vi "1553B_帧解析_v4_27.vi"(8 "ZhuBeiFen?":string="Zhufen_period", 9 "Counter":u64, 11 "数组":u8[](array[numeric])) -> (1 "连接的字符串":string, 3 "输出簇":T1)   [LabVIEW 2012]
uses:
  <vilib>/GPower/VIRegister/Library/Convert/ToU16.vi
  <vilib>/GPower/VIRegister/Library/SubVIs/FindRegisterData.vi
  <vilib>/GPower/VIRegister/Library/SubVIs/ReadSub.vi
  <vilib>/GPower/VIRegister/Library/QManager/GetRegisterData.vi
  <vilib>/GPower/Error/Library/SetError.vi
  <vilib>/GPower/Error/Library/FilterCodes.vi
  <vilib>/GPower/Error/Library/Filter/FilterMulti.vi
  <vilib>/GPower/VIRegister/Library/QManager/QManagerAction.vi
  <vilib>/GPower/Error/Library/ErrorType.vi
  <vilib>/GPower/Error/Library/SplitAppended.vi
  <vilib>/GPower/Error/Library/SubVIs/ExplanationToError.vi
  <vilib>/GPower/VIRegister/Library/QManager/GetQName.vi
  <vilib>/GPower/VIRegister/Library/QManager/StartQManager.vi
  <vilib>/Utility/error.llb/Trim Whitespace.vi
  <vilib>/dlg_ctls.llb/Space Constant.vi
  <vilib>/Utility/error.llb/Error Code Database.vi
  <vilib>/GPower/Error/Library/SubVIs/SetStatus.vi
  <vilib>/GPower/Error/Library/AppendErrors.vi
  <vilib>/GPower/Error/Library/Append/AppendSingle.vi
  <vilib>/GPower/VIRegister/VIRegister.lvlib
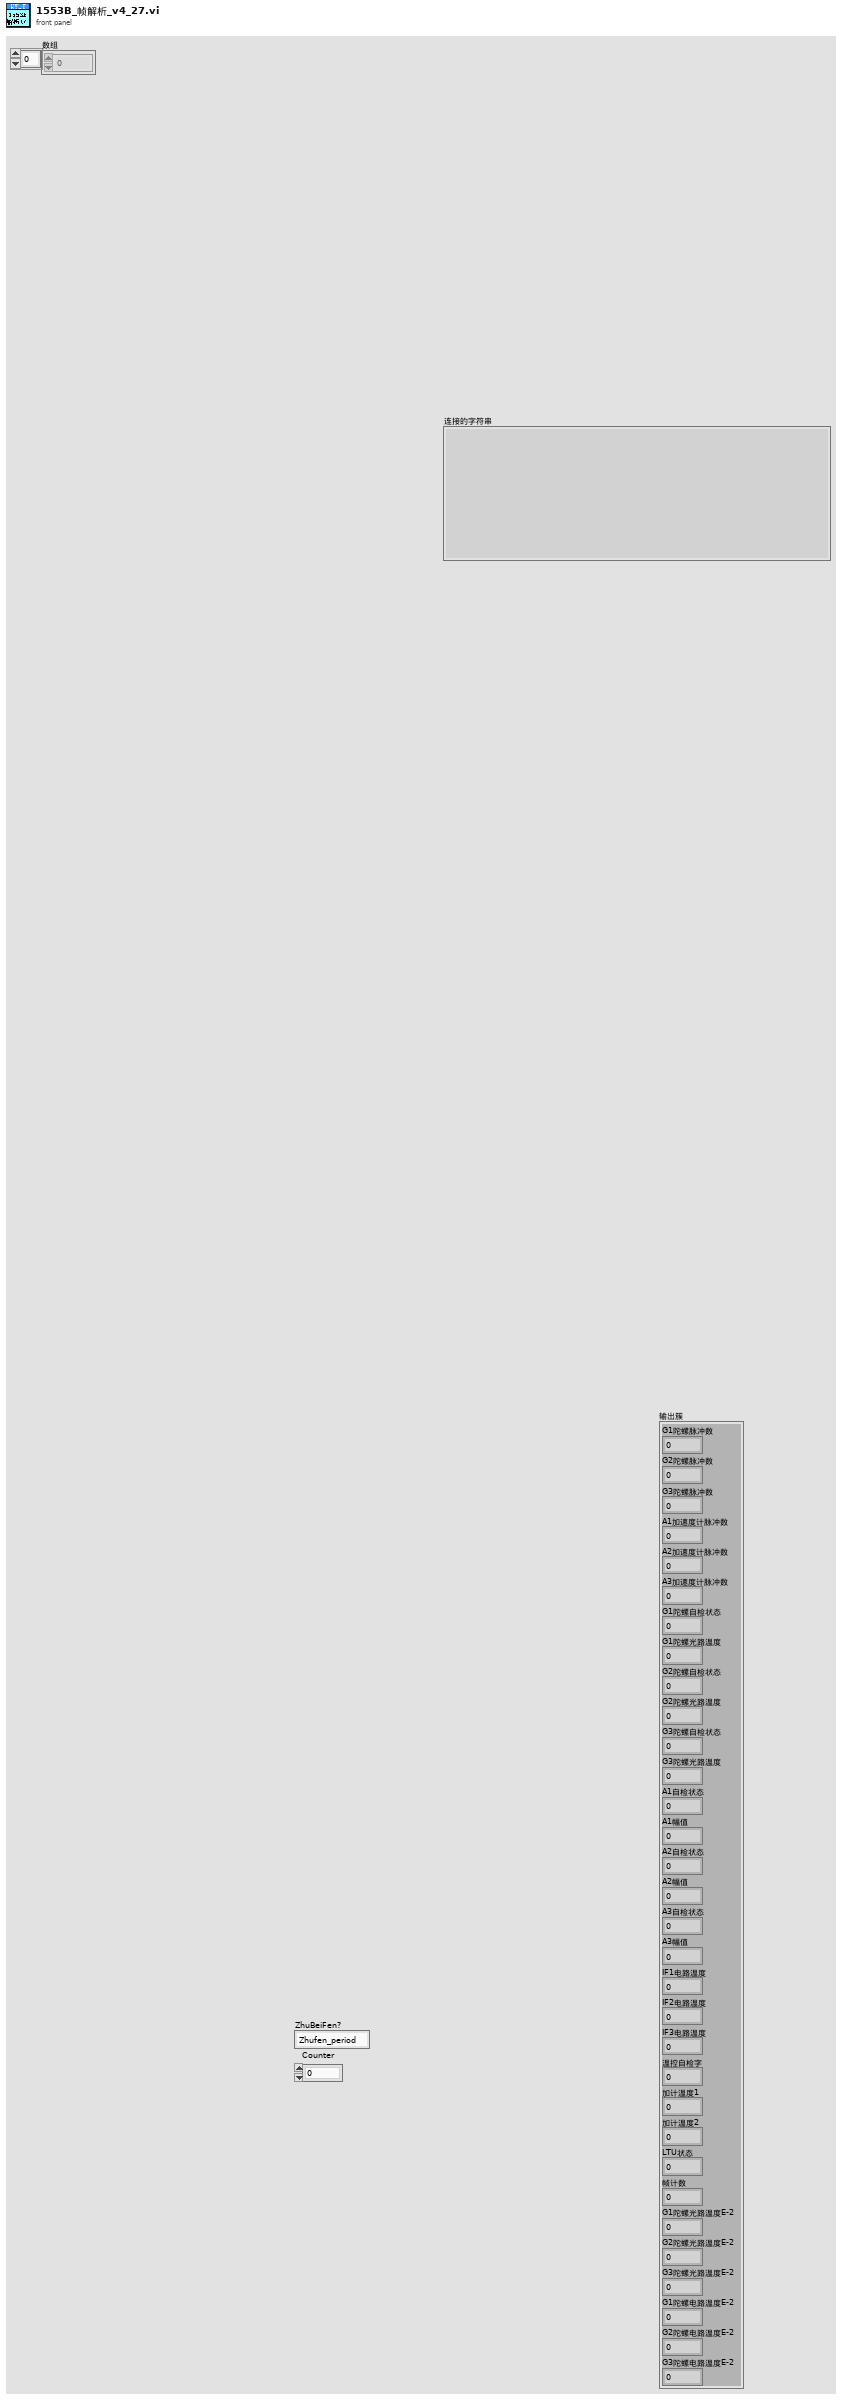
[diagram p1: front panel]
types:
  T1 = cluster{"G1陀螺脉冲数":i32, "G2陀螺脉冲数":i32, "G3陀螺脉冲数":i32, "A1加速度计脉冲数":i16, "A2加速度计脉冲数":i16, "A3加速度计脉冲数":i16, "G1陀螺自检状态":u8, "G1陀螺光路温度":i8, "G2陀螺自检状态":u8, "G2陀螺光路温度":i8, "G3陀螺自检状态":u8, "G3陀螺光路温度":i8, "A1自检状态":u8, "A1幅值":u8, "A2自检状态":u8, "A2幅值":u8, "A3自检状态":u8, "A3幅值":u8, "IF1电路温度":i8, "IF2电路温度":i8, "IF3电路温度":i8, "温控自检字":u8, "加计温度1":i16, "加计温度2":i16, "LTU状态":u8, "帧计数":u8, "G1陀螺光路温度E-2":i16, "G2陀螺光路温度E-2":i16, "G3陀螺光路温度E-2":i16, "G1陀螺电路温度E-2":i16, "G2陀螺电路温度E-2":i16, "G3陀螺电路温度E-2":i16}
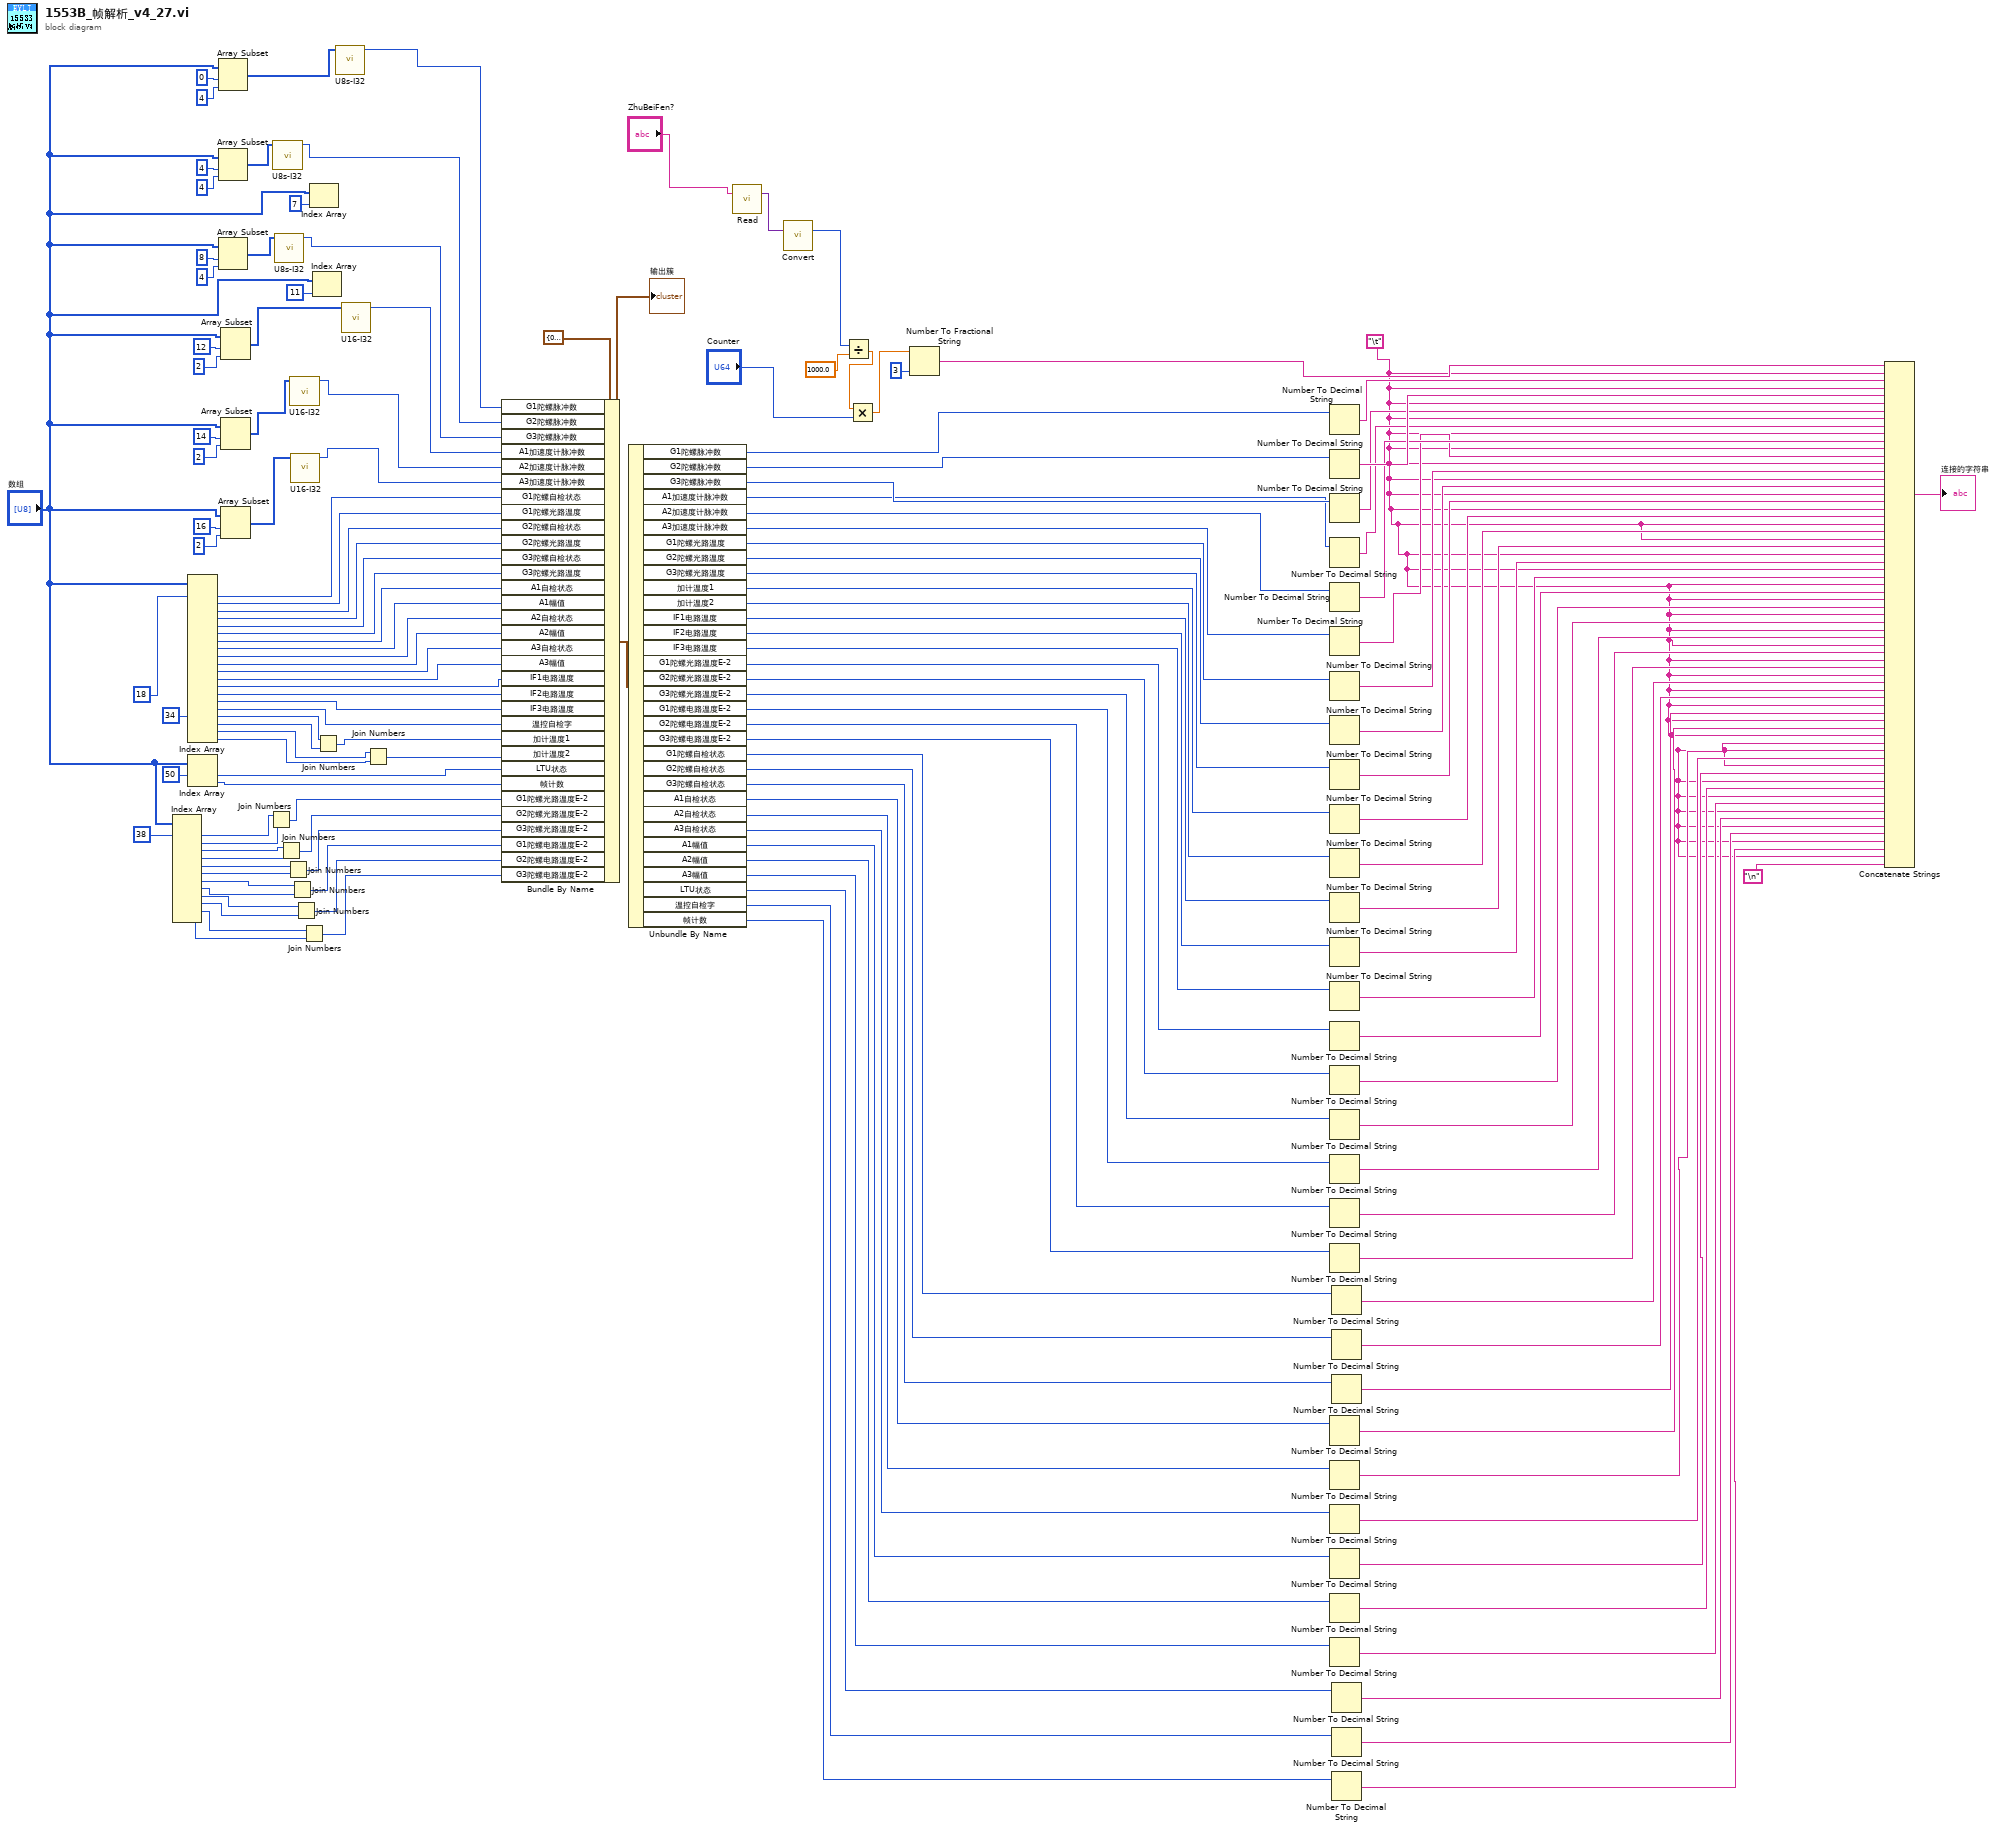
[diagram p0: block diagram]
diagram:
  w3 = "\t"
  n1 = Index Array(array="数组", index #1=38 ("索引")) -> (element #1=w34:u8, element #2=w33:u8, element #3=w31:u8, element #4=w30:u8, element #5=w28:u8, element #6=w27:u8, element #7=w25:u8, element #8=w24:u8, element #9=w20:u8, element #10=w19:u8, element #11=w18:u8, element #12=w17:u8)  [unwired: 11 in]
  n2 = Index Array(array="数组", index #1=18 ("索引"), index #17=34 ("索引")) -> (element #1=w138:u8, element #2=w78:u8, element #3=w137:u8, element #4=w136:u8, element #5=w77:u8, element #6=w76:u8, element #7=w75:u8, element #8=w74:u8, element #9=w73:u8, element #10=w72:u8, element #11=w71:u8, element #12=w70:u8, element #13=w69:u8, element #14=w68:u8, element #15=w67:u8, element #16=w66:u8, element #17=w65:u8, element #18=w63:u8, element #19=w61:u8, element #20=w60:u8)  [unwired: 18 in]
  n3 = Index Array(array="数组", index #1=50 ("索引")) -> (element #1=w58:u8, element #2=w37:u8)  [unwired: 1 in]
  n4 = Array Subset(array="数组", index=0 ("索引"), length=u8 4 ("新元素/子数组")) -> (w133:u8[])
  n5 = Array Subset(array="数组", index=4 ("索引"), length=u8 4 ("新元素/子数组")) -> (w131:u8[])
  n6 = Array Subset(array="数组", index=8 ("索引"), length=u8 4 ("新元素/子数组")) -> (w128:u8[])
  n7 = Array Subset(array="数组", index=12 ("索引"), length=u8 2 ("新元素/子数组")) -> (w127:u8[])
  n8 = Array Subset(array="数组", index=14 ("索引"), length=u8 2 ("新元素/子数组")) -> (w125:u8[])
  n9 = Array Subset(array="数组", index=16 ("索引"), length=u8 2 ("新元素/子数组")) -> (w123:u8[])
  n10 = Join Numbers(hi=w34, lo=w33) -> ((hi.lo)=w32:u16)
  n11 = call "U8s-I32.vi"("数组"=w131) -> ("I32转换"=w130:i32)  [unwired: 10 in]
  n12 = call "U8s-I32.vi"("数组"=w128) -> ("I32转换"=w129:i32)  [unwired: 10 in]
  n13 = Join Numbers(hi=w31, lo=w30) -> ((hi.lo)=w29:u16)
  n14 = Join Numbers(hi=w28, lo=w27) -> ((hi.lo)=w26:u16)
  n15 = Join Numbers(hi=w25, lo=w24) -> ((hi.lo)=w23:u16)
  n16 = call "U16-I32.vi"("数组"=w125) -> ("I32转换"=w124:i16)  [unwired: 10 in]
  n17 = call "U16-I32.vi"("数组"=w123) -> ("I32转换"=w122:i16)  [unwired: 10 in]
  n18 = Join Numbers(hi=w20, lo=w19) -> ((hi.lo)=w22:u16)
  n19 = Join Numbers(hi=w18, lo=w17) -> ((hi.lo)=w21:u16)
  n20 = Index Array(array="数组", index=7 ("索引")) -> ()  [unwired: 1 out]
  n21 = Index Array(array="数组", index=11 ("索引")) -> ()  [unwired: 1 out]
  n22 = Join Numbers(hi=w65, lo=w63) -> ((hi.lo)=w64:u16)
  n23 = call "U8s-I32.vi"("数组"=w133) -> ("I32转换"=w132:i32)  [unwired: 10 in]
  n24 = call "U16-I32.vi"("数组"=w127) -> ("I32转换"=w126:i16)  [unwired: 10 in]
  n25 = Join Numbers(hi=w61, lo=w60) -> ((hi.lo)=w62:u16)
  n26 = Bundle By Name(cluster=T1 {"G1陀螺脉冲数"=0, "G2陀螺脉冲数"=0, "G3陀螺脉冲数"=0, "A1加速度计脉冲数"=0, "A2加速度计脉冲数"=0, "A3加速度计脉冲数"=0, "G1陀螺自检状态"=0, "G1陀螺光路温度"=0, "G2陀螺自检状态"=0, "G2陀螺光路温度"=0, "G3陀螺自检状态"=0, "G3陀螺光路温度"=0, "A1自检状态"=0, "A1幅值"=0, "A2自检状态"=0, "A2幅值"=0, "A3自检状态"=0, "A3幅值"=0, "IF1电路温度"=0, "IF2电路温度"=0, "IF3电路温度"=0, "温控自检字"=0, "加计温度1"=0, "加计温度2"=0, "LTU状态"=0, "帧计数"=0, "G1陀螺光路温度E-2"=0, "G2陀螺光路温度E-2"=0, "G3陀螺光路温度E-2"=0, "G1陀螺电路温度E-2"=0, "G2陀螺电路温度E-2"=0, "G3陀螺电路温度E-2"=0} ("输入簇"), "G1陀螺脉冲数"=w132, "G2陀螺脉冲数"=w130, "G3陀螺脉冲数"=w129, "A1加速度计脉冲数"=w126, "A2加速度计脉冲数"=w124, "A3加速度计脉冲数"=w122, "G1陀螺自检状态"=w138, "G1陀螺光路温度"=w78, "G2陀螺自检状态"=w137, "G2陀螺光路温度"=w136, "G3陀螺自检状态"=w77, "G3陀螺光路温度"=w76, "A1自检状态"=w75, "A1幅值"=w74, "A2自检状态"=w73, "A2幅值"=w72, "A3自检状态"=w71, "A3幅值"=w70, "IF1电路温度"=w69, "IF2电路温度"=w68, "IF3电路温度"=w67, "温控自检字"=w66, "加计温度1"=w64, "加计温度2"=w62, "LTU状态"=w58, "帧计数"=w37, "G1陀螺光路温度E-2"=w32, "G2陀螺光路温度E-2"=w29, "G3陀螺光路温度E-2"=w26, "G1陀螺电路温度E-2"=w23, "G2陀螺电路温度E-2"=w22, "G3陀螺电路温度E-2"=w21) -> (w16:T1)
  "输出簇" <- w16
  n27 = Unbundle By Name(w16) -> ("G1陀螺脉冲数"=w121:i32, "G2陀螺脉冲数"=w120:i32, "G3陀螺脉冲数"=w119:i32, "A1加速度计脉冲数"=w118:i16, "A2加速度计脉冲数"=w117:i16, "A3加速度计脉冲数"=w116:i16, "G1陀螺光路温度"=w115:i8, "G2陀螺光路温度"=w114:i8, "G3陀螺光路温度"=w113:i8, "加计温度1"=w112:i16, "加计温度2"=w111:i16, "IF1电路温度"=w110:i8, "IF2电路温度"=w109:i8, "IF3电路温度"=w108:i8, "G1陀螺光路温度E-2"=w15:i16, "G2陀螺光路温度E-2"=w14:i16, "G3陀螺光路温度E-2"=w13:i16, "G1陀螺电路温度E-2"=w12:i16, "G2陀螺电路温度E-2"=w11:i16, "G3陀螺电路温度E-2"=w10:i16, "G1陀螺自检状态"=w87:u8, "G2陀螺自检状态"=w86:u8, "G3陀螺自检状态"=w85:u8, "A1自检状态"=w57:u8, "A2自检状态"=w56:u8, "A3自检状态"=w55:u8, "A1幅值"=w54:u8, "A2幅值"=w53:u8, "A3幅值"=w52:u8, "LTU状态"=w51:u8, "温控自检字"=w50:u8, "帧计数"=w49:u8)
  n28 = call <vilib>:"Read.vi"("Register name"="ZhuBeiFen?") -> ("Register value"=w81:variant)  [unwired: 11 in, 3 out]
  n29 = call-poly <vilib>:"Convert.vi"("Register value in"=w81) -> ("Register value out"=w80:u16)  [unwired: 13 in, 1 out]
  n30 = Divide(x=w80, y=sgl 1000.0) -> (x/y=w89:sgl)
  n31 = Multiply(x=w89, y="Counter") -> (x*y=w88:sgl)
  n32 = Number To Fractional String(number=w88, precision (6)=i16 3 ("精度(6)")) -> (F-format string=w90:string)  [unwired: 2 in]
  n33 = Number To Decimal String(number=w121) -> (decimal integer string=w107:string)  [unwired: 1 in]
  n34 = Number To Decimal String(number=w120) -> (decimal integer string=w106:string)  [unwired: 1 in]
  n35 = Number To Decimal String(number=w119) -> (decimal integer string=w105:string)  [unwired: 1 in]
  n36 = Number To Decimal String(number=w118) -> (decimal integer string=w104:string)  [unwired: 1 in]
  n37 = Number To Decimal String(number=w117) -> (decimal integer string=w103:string)  [unwired: 1 in]
  n38 = Number To Decimal String(number=w116) -> (decimal integer string=w102:string)  [unwired: 1 in]
  n39 = Number To Decimal String(number=w115) -> (decimal integer string=w101:string)  [unwired: 1 in]
  n40 = Number To Decimal String(number=w114) -> (decimal integer string=w100:string)  [unwired: 1 in]
  n41 = Number To Decimal String(number=w113) -> (decimal integer string=w99:string)  [unwired: 1 in]
  n42 = Number To Decimal String(number=w112) -> (decimal integer string=w98:string)  [unwired: 1 in]
  n43 = Number To Decimal String(number=w111) -> (decimal integer string=w97:string)  [unwired: 1 in]
  n44 = Number To Decimal String(number=w110) -> (decimal integer string=w96:string)  [unwired: 1 in]
  n45 = Number To Decimal String(number=w109) -> (decimal integer string=w95:string)  [unwired: 1 in]
  n46 = Number To Decimal String(number=w108) -> (decimal integer string=w94:string)  [unwired: 1 in]
  n47 = Number To Decimal String(number=w15) -> (decimal integer string=w9:string)  [unwired: 1 in]
  n48 = Number To Decimal String(number=w14) -> (decimal integer string=w8:string)  [unwired: 1 in]
  n49 = Number To Decimal String(number=w13) -> (decimal integer string=w7:string)  [unwired: 1 in]
  n50 = Number To Decimal String(number=w12) -> (decimal integer string=w6:string)  [unwired: 1 in]
  n51 = Number To Decimal String(number=w11) -> (decimal integer string=w5:string)  [unwired: 1 in]
  n52 = Number To Decimal String(number=w10) -> (decimal integer string=w4:string)  [unwired: 1 in]
  n53 = Number To Decimal String(number=w57) -> (decimal integer string=w48:string)  [unwired: 1 in]
  n54 = Number To Decimal String(number=w56) -> (decimal integer string=w47:string)  [unwired: 1 in]
  n55 = Number To Decimal String(number=w55) -> (decimal integer string=w46:string)  [unwired: 1 in]
  n56 = Number To Decimal String(number=w54) -> (decimal integer string=w45:string)  [unwired: 1 in]
  n57 = Number To Decimal String(number=w53) -> (decimal integer string=w44:string)  [unwired: 1 in]
  n58 = Number To Decimal String(number=w52) -> (decimal integer string=w43:string)  [unwired: 1 in]
  n59 = Number To Decimal String(number=w87) -> (decimal integer string=w84:string)  [unwired: 1 in]
  n60 = Number To Decimal String(number=w86) -> (decimal integer string=w83:string)  [unwired: 1 in]
  n61 = Number To Decimal String(number=w85) -> (decimal integer string=w82:string)  [unwired: 1 in]
  n62 = Number To Decimal String(number=w51) -> (decimal integer string=w42:string)  [unwired: 1 in]
  n63 = Number To Decimal String(number=w50) -> (decimal integer string=w41:string)  [unwired: 1 in]
  n64 = Number To Decimal String(number=w49) -> (decimal integer string=w40:string)  [unwired: 1 in]
  n65 = Concatenate Strings(w90, w3, w107, w3, w106, w3, w105, w3, w104, w3, w103, w3, w102, w3, w101, w3, w100, w3, w99, w3, w98, w3, w97, w3, w96, w3, w95, w3, w94, w3, w9, w3, w8, w3, w7, w3, w6, w3, w5, w3, w4, w3, w84, w3, w83, w3, w82, w3, w48, w3, w47, w3, w46, w3, w45, w3, w44, w3, w43, w3, w42, w3, w41, w3, w40, w3, "\n") -> (→"连接的字符串":string)
